vi "DelayTime.vi"(1 "Detector Select":enum32{"4 Detectors", "8 Detectors"}(radio)=enum."8 Detectors") -> (0 "Delaytime":sgl[](array[numeric]))   [LabVIEW 2014]
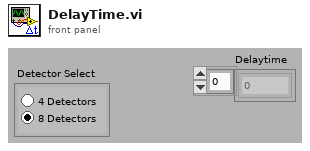
[diagram p1: front panel]
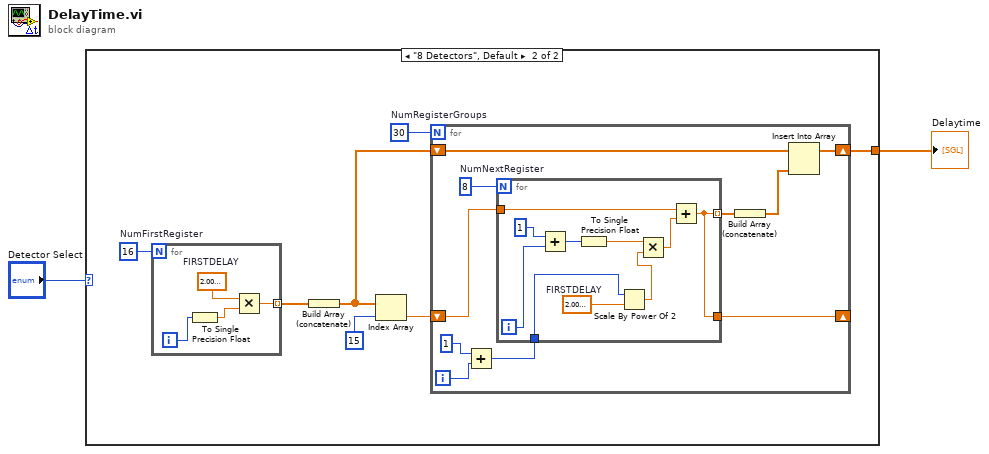
[diagram p0: block diagram]
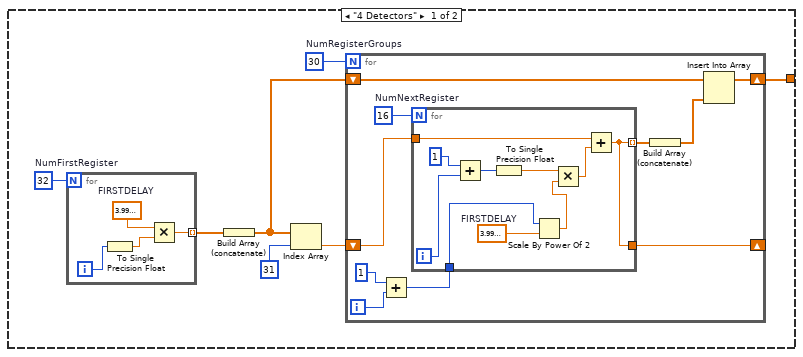
[diagram p2: hidden frame]
diagram:
  n1 = case shown="\"8 Detectors\", Default" "Detector Select" {
    tunnel: [w3 w34] -> w1
    frame "4 Detectors" {
      w5 = 30  # NumRegisterGroups
      w4 = 32  # NumFirstRegister
      n2 = for {
        N: w4 -> [_]
        tunnel: [w31] -> w6 mode=indexing
        i -> [w30]
        w33 = sgl 4e-08  # FIRSTDELAY
        n3 = To Single Precision Float(number=w30) -> (single precision float=w32:sgl)
        n4 = Multiply(x=w33, y=w32) -> (x*y=w31:sgl)
      }
      n5 = Build Array (concatenate)(w6) -> (w8:sgl[])
      n6 = Index Array(array=w8, index=31) -> (element=w9:sgl)
      n7 = for {
        N: w5 -> [_]
        shift-right: [w12] -> _
        shift-left: w9 -> [w16]
        shift-right: [w13] -> w3
        shift-left: w8 -> [w14]
        i -> [w10]
        w19 = 16  # NumNextRegister
        n8 = Add(x=1, y=w10) -> (x+y=w17:i32)
        n9 = for {
          N: w19 -> [_]
          tunnel: [w23] -> w12
          tunnel: w17 -> [w28]
          tunnel: [w23] -> w15 mode=indexing
          tunnel: w16 -> [w24]
          i -> [w21]
          w29 = sgl 4e-08  # FIRSTDELAY
          n10 = Add(x=1, y=w21) -> (x+y=w22:i32)
          n11 = To Single Precision Float(number=w22) -> (single precision float=w26:sgl)
          n12 = Scale By Power Of 2(n=w28, x=w29) -> (x*2^n=w27:sgl)
          n13 = Multiply(x=w26, y=w27) -> (x*y=w25:sgl)
          n14 = Add(x=w24, y=w25) -> (x+y=w23:sgl)
        }
        n15 = Build Array (concatenate)(w15) -> (w11:sgl[])
        n16 = Insert Into Array(array=w14, new element=w11) -> (w13:sgl[])  [unwired: 1 in]
      }
    }
    frame "8 Detectors", Default {
      w36 = 30  # NumRegisterGroups
      w35 = 16  # NumFirstRegister
      n17 = for {
        N: w35 -> [_]
        tunnel: [w62] -> w37 mode=indexing
        i -> [w61]
        w64 = sgl 2e-07  # FIRSTDELAY
        n18 = To Single Precision Float(number=w61) -> (single precision float=w63:sgl)
        n19 = Multiply(x=w64, y=w63) -> (x*y=w62:sgl)
      }
      n20 = Build Array (concatenate)(w37) -> (w39:sgl[])
      n21 = Index Array(array=w39, index=15) -> (element=w40:sgl)
      n22 = for {
        N: w36 -> [_]
        shift-right: [w43] -> _
        shift-left: w40 -> [w47]
        shift-right: [w44] -> w34
        shift-left: w39 -> [w45]
        i -> [w41]
        w50 = 8  # NumNextRegister
        n23 = Add(x=1, y=w41) -> (x+y=w48:i32)
        n24 = for {
          N: w50 -> [_]
          tunnel: [w54] -> w43
          tunnel: w48 -> [w59]
          tunnel: [w54] -> w46 mode=indexing
          tunnel: w47 -> [w55]
          i -> [w52]
          w60 = sgl 2e-07  # FIRSTDELAY
          n25 = Add(x=1, y=w52) -> (x+y=w53:i32)
          n26 = To Single Precision Float(number=w53) -> (single precision float=w57:sgl)
          n27 = Scale By Power Of 2(n=w59, x=w60) -> (x*2^n=w58:sgl)
          n28 = Multiply(x=w57, y=w58) -> (x*y=w56:sgl)
          n29 = Add(x=w55, y=w56) -> (x+y=w54:sgl)
        }
        n30 = Build Array (concatenate)(w46) -> (w42:sgl[])
        n31 = Insert Into Array(array=w45, new element=w42) -> (w44:sgl[])  [unwired: 1 in]
      }
    }
  }
  "Delaytime" <- w1
